vi "Start Acquisition and Logging.vi"(8 "error in (no error)":errorcluster, 11 "Acquisition and Logging Configuration":T1={"Data Rate"=1, "Samples per Read"=0, "Number of Reads to Save"=0, "Data File Name"="", "TDMS Properties"=[], "Number of Channels"=4, "Channel Scale Array"=[0.0, 0.0, 0.0, 0.0, 1.0, 1.0, 1.0, 1.0], "Channel Names"=[], "Trigger - RMS Value"=0.0, "Trigger - Channel"=0, "Trigger - Time (Minute)"=0} {"Data Rate" items=["51.200 kS/s (NI 9234)"=1, "25.600 kS/s (NI 9234)"=2, "17.067 kS/s (NI 9234)"=3, "12.800 kS/s (NI 9234)"=4, "10.240 kS/s (NI 9234)"=5, "8.533 kS/s (NI 9234)"=6, "7.314 kS/s (NI 9234)"=7, "6.400 kS/s (NI 9234)"=8, "5.689 kS/s (NI 9234)"=9, "5.120 kS/s (NI 9234)"=10, "4.654 kS/s (NI 9234)"=11, "4.267 kS/s (NI 9234)"=12, "3.938 kS/s (NI 9234)"=13, "3.657 kS/s (NI 9234)"=14, "3.413 kS/s (NI 9234)"=15, "3.200 kS/s (NI 9234)"=16, "3.012 kS/s (NI 9234)"=17, "2.845 kS/s (NI 9234)"=18, "2.695 kS/s (NI 9234)"=19, "2.560 kS/s (NI 9234)"=20, "2.438 kS/s (NI 9234)"=21, "2.328 kS/s (NI 9234)"=22, "2.226 kS/s (NI 9234)"=23, "2.133 kS/s (NI 9234)"=24, "2.048 kS/s (NI 9234)"=25, "1.969 kS/s (NI 9234)"=26, "1.896 kS/s (NI 9234)"=27, "1.829 kS/s (NI 9234)"=28, "1.765 kS/s (NI 9234)"=29, "1.707 kS/s (NI 9234)"=30, "1.652 kS/s (NI 9234)"=31]}) -> (0 "error out":errorcluster, 1 "Wait on IRQ Timeout?":bool, 2 "Total Buffer Size":i32, 3 "FPGA VI Reference Out":T4)   [LabVIEW 2015]
uses:
  <vilib>/rvi/interface/nirviMethod/nirviMethod.xnode
  <vilib>/rvi/interface/nirviReadWriteControl/nirviReadWriteControl.xnode
  <vilib>/rvi/errors/niLvFpgaMergeErrorWithErrorCode.vi
  <vilib>/rvi/interface/nirviOpenFPGA/nirviOpenFPGA.xnode
  <vilib>/FPGAPlugInAG/Dynamic/niLvFpga_Reset_Dynamic.vi
  <vilib>/FPGAPlugInAG/Dynamic/niLvFpga_Run_Dynamic.vi
  <vilib>/rvi/interface/nirviMethod/StockFPGA_InlinedMethodWaitForSingleIRQ.vi
  <vilib>/FPGAPlugInAG/Dynamic/niLvFpga_WaitOnIrq_Dynamic.vi
  <vilib>/FPGAPlugInAG/Dynamic/niLvFpga_AcknowledgeIrq_Dynamic.vi
  NiFpgaLv.dll
  <vilib>/Utility/error.llb/Error Cluster From Error Code.vi
  <vilib>/rvi/interface/Simulation/niFpgaSimulationCallBeginRW.vi
  <vilib>/rvi/errors/niLvFpgaAdjustHostInterfaceError.vi
  <vilib>/FPGAPlugInAG/Dynamic/niLvFpga_ConfigureFifo_Dynamic.vi
  <vilib>/FPGAPlugInAG/Dynamic/niLvFpga_StartFifo_Dynamic.vi
  FPGA Bitfiles/CrioFPGA-RT-NSCo_FPGATarget2_FPGAMain2Modules_4cECY-5hqZ0.lvbitx
  FPGA Main_2Modules.vi
  <vilib>/FPGAPlugInAG/cRIO-9112/niLvFpga_Open_cRIO-9112.vi
  <vilib>/rvi/interface/common/dynamic/niFpgaDynamicAddResources.vi
  controls/FPGA VI Reference.ctl
  controls/Acquisition and Logging Configuration.ctl
  <vilib>/LabVIEW Targets/FPGA/cRIO/shared/nicrio_ModuleControls/nicrio_cRIO-9234_DataRatesRing2.ctl
  controls/TDMS Properties.ctl
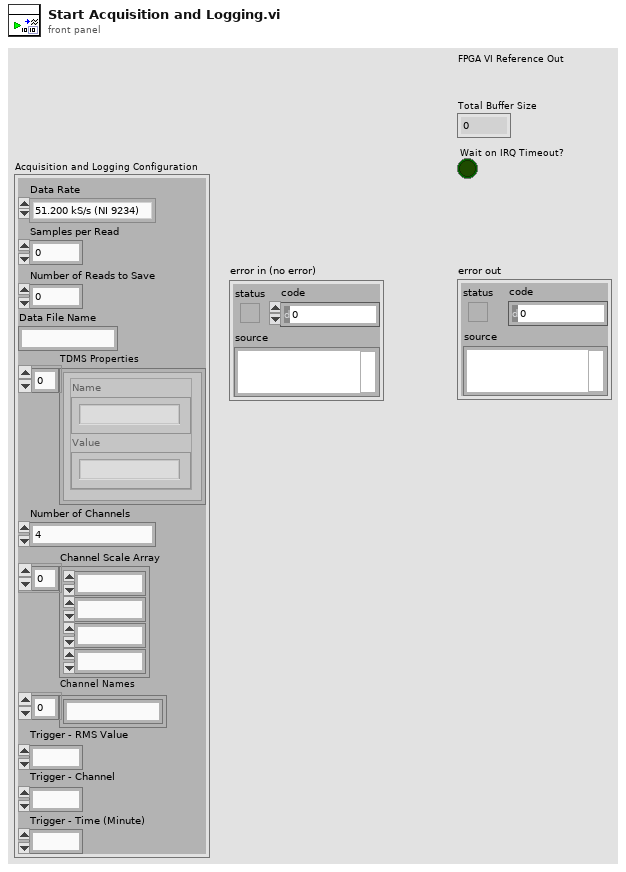
[diagram p1: front panel]
types:
  T1 = typedef "Acquisition and Logging Configuration.ctl" = cluster{"Data Rate":T2, "Samples per Read":i32, "Number of Reads to Save":i32, "Data File Name":string, "TDMS Properties":T3[], "Number of Channels":i32, "Channel Scale Array":fxp<+,24,12>[], "Channel Names":string[], "Trigger - RMS Value":dbl, "Trigger - Channel":i32, "Trigger - Time (Minute)":i32}
  T2 = typedef "nicrio_cRIO-9234_DataRatesRing2.ctl" = u8
  T3 = typedef "TDMS Properties.ctl" = cluster{"Name":string, "Value":string}
  T4 = typedef "FPGA VI Reference.ctl" = refnum<k20>
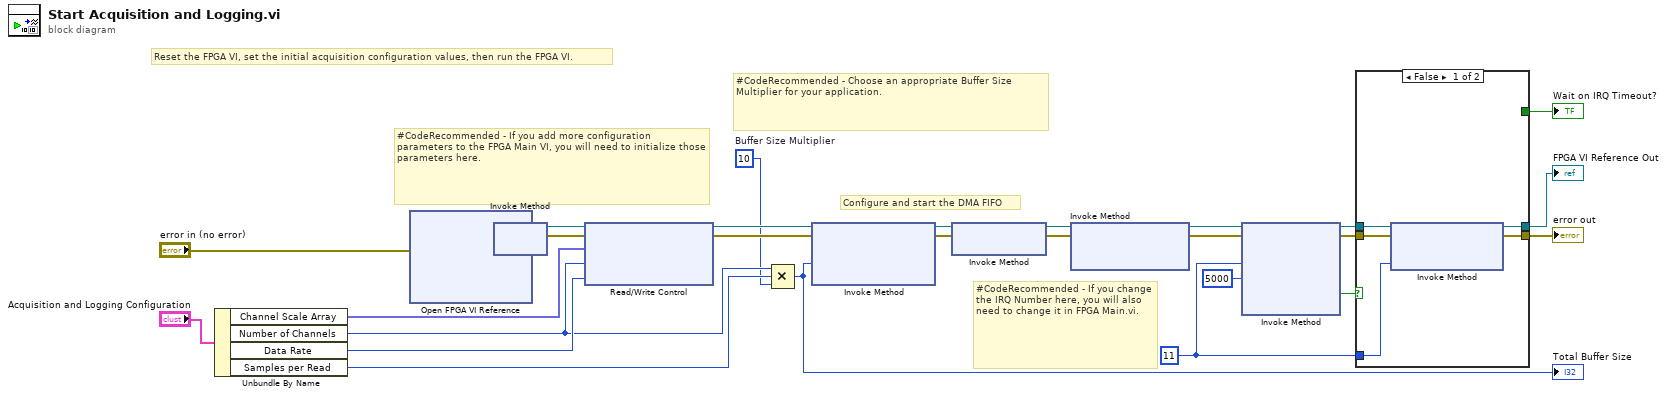
[diagram p0: block diagram]
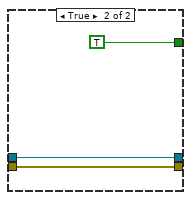
[diagram p2: hidden frame]
diagram:
  w5 = 11
  w6 = 10  # Buffer Size Multiplier
  # "#CodeRecommended - If you change the IRQ Number here, you will also need to change it in FPGA Main.vi."
  # "#CodeRecommended - Choose an appropriate Buffer Size Multiplier for your application."
  # "Configure and start the DMA FIFO"
  # "#CodeRecommended - If you add more configuration parameters to the FPGA Main VI, you will need to initialize those parameters here."
  # "Reset the FPGA VI, set the initial acquisition configuration values, then run the FPGA VI."
  n1 = Unbundle By Name("Acquisition and Logging Configuration") -> ("Channel Scale Array"=w18:fxp<+,24,12>[], "Number of Channels"=w9:i32, "Data Rate"=w17:T2, "Samples per Read"=w8:i32)
  n2 = xnode "Open FPGA VI Reference"("error in"="error in (no error)") -> ("FPGA VI Reference Out"=w4:refnum<k20>, "error out"=w3:errorcluster)  [unwired: 1 in]
  n3 = xnode "Invoke Method"("FPGA VI Reference In"=w4, "error in"=w3) -> ("FPGA VI Reference Out"=w26:refnum<k20>, "error out"=w25:errorcluster)
  n4 = xnode "Read/Write Control"("FPGA VI Reference In"=w26, "error in"=w25, "Channel Scale Array"=w18, "Number of Channels"=w9, "Data Rate"=w17) -> ("FPGA VI Reference Out"=w11:refnum<k20>, "error out"=w10:errorcluster)
  n5 = Compound Arithmetic op=MULTIPLY(w9, w8, w6) -> (w7:i32)
  "Total Buffer Size" <- w7
  n6 = xnode "Invoke Method"("FPGA VI Reference In"=w11, "error in"=w10, "Requested Depth"=w7) -> ("FPGA VI Reference Out"=w14:refnum<k20>, "error out"=w15:errorcluster)  [unwired: 1 out]
  n7 = xnode "Invoke Method"("FPGA VI Reference In"=w14, "error in"=w15) -> ("FPGA VI Reference Out"=w12:refnum<k20>, "error out"=w13:errorcluster)
  n8 = xnode "Invoke Method"("FPGA VI Reference In"=w12, "error in"=w13) -> ("FPGA VI Reference Out"=w27:refnum<k20>, "error out"=w28:errorcluster)  [unwired: 1 in]
  n9 = xnode "Invoke Method"("FPGA VI Reference In"=w27, "error in"=w28, "IRQ Number(s)"=w5, "Timeout (ms)"=5000) -> ("FPGA VI Reference Out"=w19:refnum<k20>, "error out"=w20:errorcluster, "Timed Out"=w22:bool)  [unwired: 1 out]
  n10 = case shown="False" w22 {
    tunnel: w19 -> [w33 w34]
    tunnel: w20 -> [w32 w36]
    tunnel: [w31 w36] -> w23
    tunnel: w5 -> [w30 _]
    tunnel: [_ TRUE] -> w24
    tunnel: [w29 w34] -> w1
    frame False {
      n11 = xnode "Invoke Method"("FPGA VI Reference In"=w33, "error in"=w32, "IRQ Number(s)"=w30) -> ("FPGA VI Reference Out"=w29:refnum<k20>, "error out"=w31:errorcluster)
    }
    frame True {
    }
  }
  "FPGA VI Reference Out" <- w1
  "Wait on IRQ Timeout?" <- w24
  "error out" <- w23
